vi "Integrate Wheels.vi"(11 "change in time s":dbl) -> (3 "XY Graph":cluster{dbl[], dbl[]}(graph))   [LabVIEW 2016]
uses:
  Gyro/MyRIO/VI/Public/MPU6050 Read Z Rotation.vi
  Globals/Position.vi
  Globals/Gyro.vi
  Gyro/MyRIO/VI/Private/MPU6050 Read Rotation Data.vi
panel:
  in  "Gyro Trust":dbl=1.0
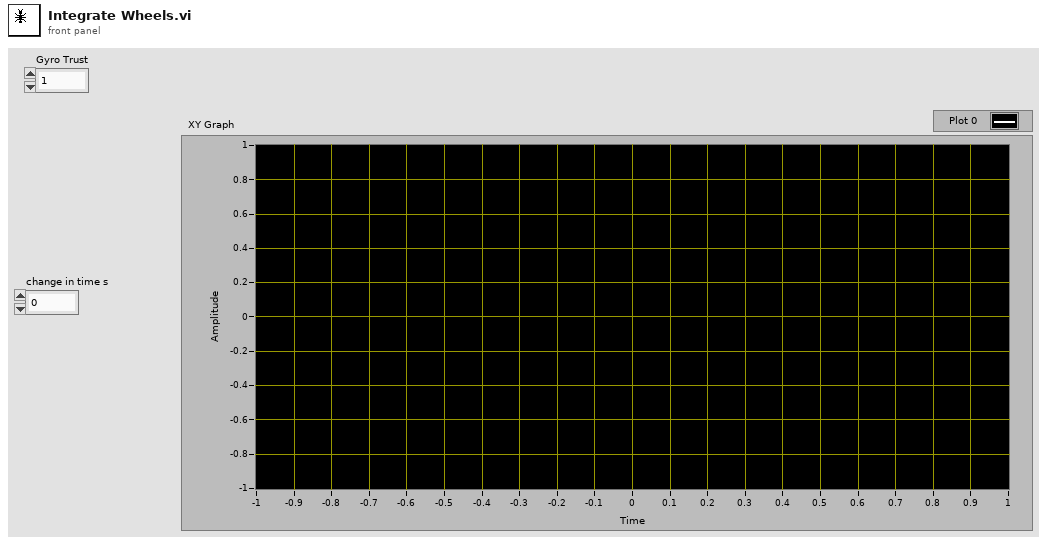
[diagram p1: front panel]
types:
  T1 = typedef "I2C.lvlib/I2C Reference.ctl" = cluster{"myRIO Reference":T2, "I2C Channels Enum":T6, "I2C Configuration":T7}
  T2 = typedef "myRIO Generic Hardware Reference.ctl" = cluster{"myRIO Model":T3, "myRIO Hardware Reference":T4}
  T3 = typedef "Hardware Version Enum.ctl" = enum16{"Unknown", "myRIO-1900", "myRIO-1950", "roboRIO", "NI ELVIS RIO CM"}
  T4 = typedef "myRIO v1.0 Reference.ctl" = cluster{"Generic FPGA Reference":T5, "Allow multiple opens":bool}
  T5 = typedef "Generic FPGA Reference.ctl" = refnum<k20>
  T6 = typedef "I2C Channels Enum.ctl" = enum16{"Not Connected", "A/I2C", "B/I2C", "I2C/I2C"}
  T7 = typedef "I2C.lvlib/I2C Configuration.ctl" = cluster{"I2C Transfer Rate":T8}
  T8 = typedef "I2C.lvlib/I2C Transfer Rate.ctl" = enum16{"Standard mode (100 kbps)", "Fast mode (400 kbps)"}
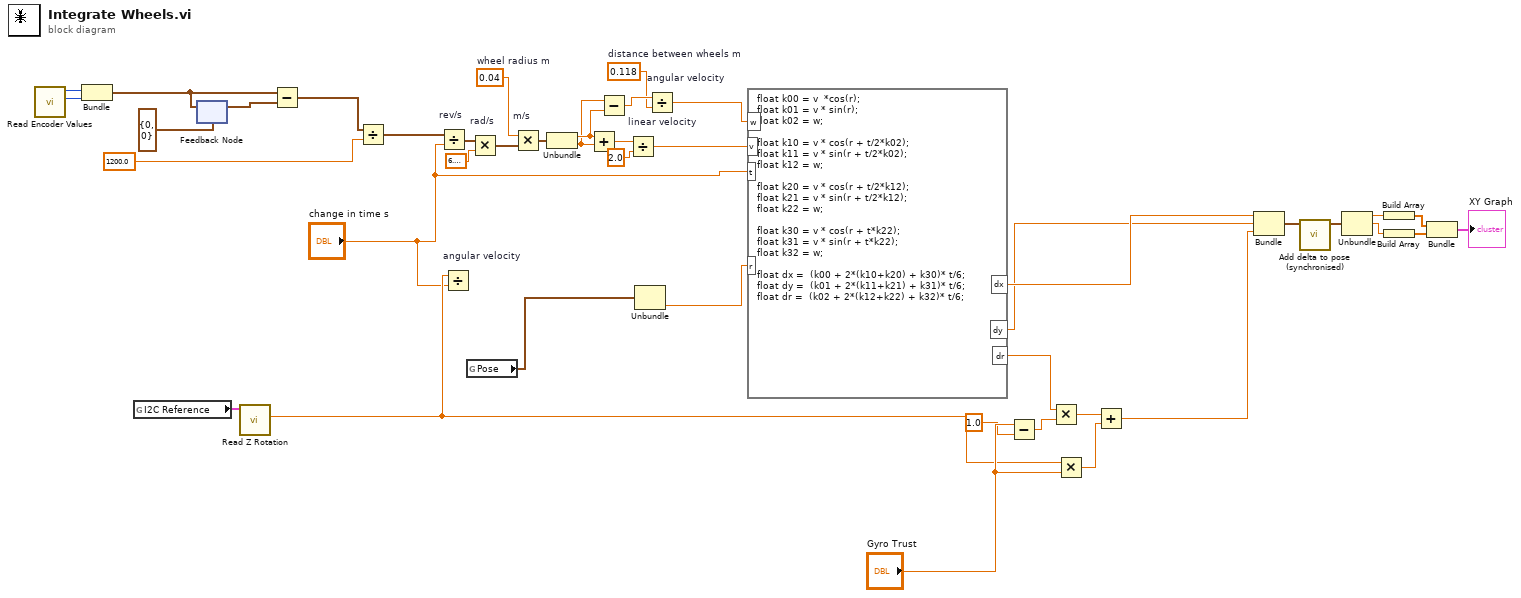
[diagram p0: block diagram]
diagram:
  w32 = 0.118  # distance between wheels m
  w40 = 0.04  # wheel radius m
  n1 = call "Read Encoder Values.vi"() -> ("Right Value"=w10:i32, "Left  Value"=w9:i32)  [unwired: 10 in]
  n2 = Bundle("Left  Value"=w9, "Right Value"=w10) -> (w12:cluster{"Left  Value":i32, "Right Value":i32})  [unwired: 1 in]
  n3 = global read "Gyro.vi" "I2C Reference"() -> (w22:T1)
  n4 = feedback #1(cluster{"Left  Value":i32, "Right Value":i32} {"Left  Value"=0, "Right Value"=0}) -> (w13:cluster{"Left  Value":i32, "Right Value":i32})
  n5 = feedback-in #1(w12) -> ()
  n6 = call "Read Z Rotation.vi"("I2C Ref In"=w22) -> ("Z Rotation (rads)"=w5:dbl)  [unwired: 7 in, 2 out]
  n7 = Subtract(x=w12, y=w13) -> (x-y=w7:cluster{"Left  Value":i32, "Right Value":i32})
  n8 = Divide(x=w7, y=1200.0 ("Left  Value")) -> (x/y=w8:cluster{"Left  Value":dbl, "Right Value":dbl})
  n9 = Divide "rev/s"(x=w8, y="change in time s") -> (x/y=w42:cluster{"Left  Value":dbl, "Right Value":dbl})
  n10 = Divide "angular velocity"(x=w5, y="change in time s") -> ()  [unwired: 1 out]
  n11 = global read "Position.vi" "Pose"() -> (w21:cluster{"X":dbl, "Y":dbl, "Rotation":dbl})
  n12 = Multiply "rad/s"(x=w42, y=6.283185307179586) -> (x*y=w39:cluster{"Left  Value":dbl, "Right Value":dbl})
  n13 = Multiply "m/s"(x=w40, y=w39) -> (x*y=w36:cluster{"Left  Value":dbl, "Right Value":dbl})
  n14 = Unbundle(w36) -> ("Left  Value"=w35:dbl, "Right Value"=w34:dbl)
  n15 = Add(x=w35, y=w34) -> (x+y=w37:dbl)
  n16 = Subtract(x=w34, y=w35) -> (x-y=w33:dbl)
  n17 = Divide "linear velocity"(x=w37, y=2.0) -> (x/y=w31:dbl)
  n18 = Unbundle(w21) -> ("Rotation"=w30:dbl)  [unwired: 2 out]
  n19 = Divide "angular velocity"(x=w33, y=w32) -> (x/y=w3:dbl)
  n20 = formula code="float k00 = v  *cos(r);\nfloat k01 = v * sin(r);\nfloat k02 = w;\n\nfloat k10 = v * cos(r + t/2*k02);\nfloat k11 = v * sin(r + t/2*k02);\nfloat k12 = w;\n\nfloat k20 = v * cos(r + t/2*k12);\nfloat k21 = v * sin(r + t/2*k12);\nfloat k22 = w;\n\nfloat k30 = v * cos(r + t*k22);\nfloat k31 = v * sin(r + t*k22);\nfloat k32 = w;\n\nfloat dx =  (k00 + 2*(k10+k20) + k30)* t/6;\nfloat dy =  (k01 + 2*(k11+k21) + k31)* t/6;\nfloat dr =  (k02 + 2*(k12+k22) + k32)* t/6;"("w"=w3, "v"=w31, "t"="change in time s", "r"=w30) -> ("dx"=w26:dbl, "dy"=w25:dbl, "dr"=w15:dbl)
  n21 = Subtract(x="Gyro Trust", y=1.0 ("x")) -> (x-y=w18:dbl)
  n22 = Multiply(x=w15, y=w18) -> (x*y=w20:dbl)
  n23 = Multiply(x=w5, y="Gyro Trust") -> (x*y=w19:dbl)
  n24 = Add(x=w20, y=w19) -> (x+y=w6:dbl)
  n25 = Bundle(w26, w25, w6) -> (w2:cluster{dbl, dbl, dbl})  [unwired: 1 in]
  n26 = call "Add delta to pose (synchronised).vi"("Delta"=w2) -> ("New Pose"=w1:cluster{"X":dbl, "Y":dbl, "Rotation (rads)":dbl})  [unwired: 10 in]
  n27 = Unbundle(w1) -> ("X"=w24:dbl, "Y"=w23:dbl)  [unwired: 1 out]
  n28 = Build Array(w24) -> (w29:dbl[])
  n29 = Build Array(w23) -> (w28:dbl[])
  n30 = Bundle(w29, w28) -> (→"XY Graph":cluster{dbl[], dbl[]})  [unwired: 1 in]
